vi "Extract Window Origin and Size.vi"(0 "window rect":T1) -> (1 "window origin":cluster{"left":i16, "top":i16}, 2 "window size":cluster{"width":i16, "height":i16})   [LabVIEW 2011]
doc: "This VI will extract the size and origin of a window using the window rectangle as an input. This information is useful when moving or resizing a window.\n\n-------------\nMagna Package Information\n\nProduct Name: Magna Windows Utilities\nPackage File Name: Magna_Windows_Utilities\nPackage Version: 2.7.0.32\nMinimum LabVIEW Version: 11.0"
uses:
  Controls/Window Rectangle.ctl
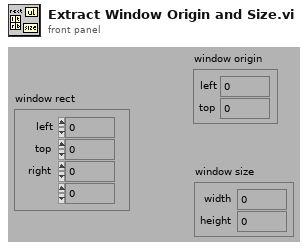
[diagram p1: front panel]
types:
  T1 = typedef "Window Rectangle.ctl" = cluster{"left":i16, "top":i16, "right":i16, "bottom":i16}
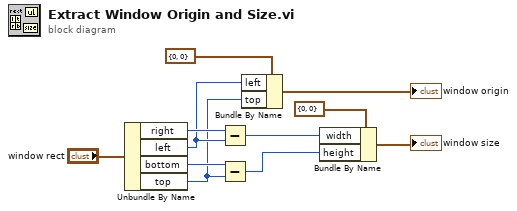
[diagram p0: block diagram]
diagram:
  n1 = Unbundle By Name("window rect") -> ("right"=w10:i16, "left"=w4:i16, "bottom"=w9:i16, "top"=w3:i16)
  n2 = Subtract(x=w10, y=w4) -> (x-y=w6:i16)
  n3 = Subtract(x=w9, y=w3) -> (x-y=w7:i16)
  n4 = Bundle By Name(cluster=cluster{"left":i16, "top":i16} {"left"=0, "top"=0} ("window origin"), "left"=w4, "top"=w3) -> (→"window origin":cluster{"left":i16, "top":i16})
  n5 = Bundle By Name(cluster=cluster{"width":i16, "height":i16} {"width"=0, "height"=0} ("window size"), "width"=w6, "height"=w7) -> (→"window size":cluster{"width":i16, "height":i16})
